vi "get experiment save on off list.vi"(0 "error out":errorcluster, 10 "MCListbox Refnum":refnum<vi>, 11 "Experiment":string) -> (3 "save status item symbols":i32[](array[numeric]))   [LabVIEW 2020]
uses:
  <userlib>/_OpenG.lib/array/array.llb/Sort 2D Array (String)__ogtk.vi
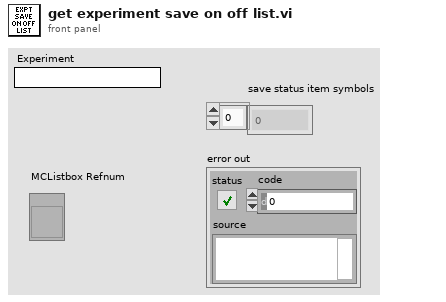
[diagram p1: front panel]
types:
  T1 = typedef "mysql_authentication.ctl" = cluster{"User":string, "Password":string, "Database":string}
  T2 = cluster{"Port":u16, "IP Address":string, "Authentication":T1}
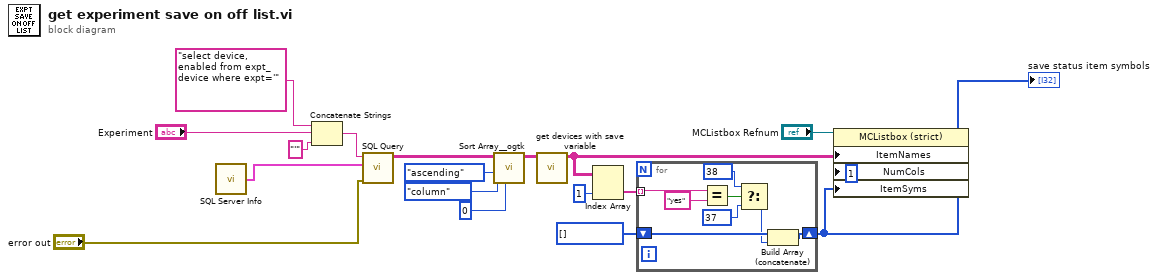
[diagram p0: block diagram]
diagram:
  n1 = call "SQL Server Info.vi"() -> ("SQL Server Info"=w7:T2)
  n2 = Concatenate Strings("select device, enabled from expt_device where expt='" ("Query"), "Experiment", "'" ("Query")) -> (w3:string)
  n3 = call "SQL Query.vi"("error in (no error)"="error out", "SQL Server Info"=w7, "Query"=w3) -> ("data"=w15:string[][])  [unwired: 7 in, 1 out]
  n4 = call-poly <userlib>:"Sort Array__ogtk.vi"("Column/Row to Sort By"=u32 0, "Sort By in"=enum16{"row", "column"}."column", "Order"=enum16{"ascending", "descending"}."ascending", "Array in"=w15) -> ("Sorted Array out"=w16:string[][])  [unwired: 4 in, 3 out]
  n5 = call "get devices with save variable.vi"("List of devices"=w16) -> ("array"=w17:string[][])  [unwired: 10 in]
  n6 = Index Array(array=w17, index (col)=1 ("disabled index (col)")) -> (element=w18:string[])  [unwired: 1 in]
  n7 = for {
    tunnel: w18 -> [w26] mode=indexing
    shift-right: [w19] -> w11
    shift-left: i32[] [] -> [w24]
    n8 = Equal?(x=w26, y="yes") -> (x = y?=w23:bool)
    n9 = Select(t=38, s=w23, f=37) -> (s? t:f=w20:i32)
    n10 = Build Array (concatenate)(w24, w20) -> (w19:i32[])
  }
  "save status item symbols" <- w11
  n11 = property on="Property Node" class="MCListbox (strict)"(reference="MCListbox Refnum", "ItemNames"=w17, "NumCols"=u32 1 ("Number of Columns"), "ItemSyms"=w11) -> ()  [unwired: 1 in, 2 out]
